vi "Send Libraries.vi"(8 "error in (no error)":errorcluster, 11 "Kasli Wrapper 2.0 in":refnum<class "Kasli Wrapper 2.0.lvclass">=refnum) -> (0 "error out":errorcluster, 3 "Kasli Wrapper 2.0 out":refnum<class "Kasli Wrapper 2.0.lvclass">)   [LabVIEW 2020, in "CIRCUS_uServices.lvlib" / "Kasli Wrapper 2.0.lvlib" / "Kasli Wrapper 2.0.lvclass"]
uses:
  Kasli Wrapper 2.0.lvclass
  TALOS/TALOS_PPL.lvlibp/Father of all uServices/Father of all uServices/Father of all uServices.lvclass
  Kasli Wrapper 2.0.lvlib
  Kasli/Kasli.lvclass
  C:/Users/marco/Documents/GitHub_Lab/CIRCUS/TALOS/TALOS_PPL.lvlibp/Ancestor/Ancestor/Ancestor.lvclass
  C:/Users/marco/Documents/GitHub_Lab/CIRCUS/TALOS/Actor Framework.lvlibp/1abvi3w/vi.lib/ActorFramework/Actor/Actor.lvclass
  C:/Users/marco/Documents/GitHub_Lab/CIRCUS/TALOS/TALOS_PPL.lvlibp/Father of all uServices/Father of all uServices/Father of all uServices.lvclass
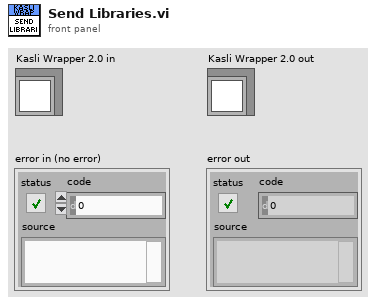
[diagram p1: front panel]
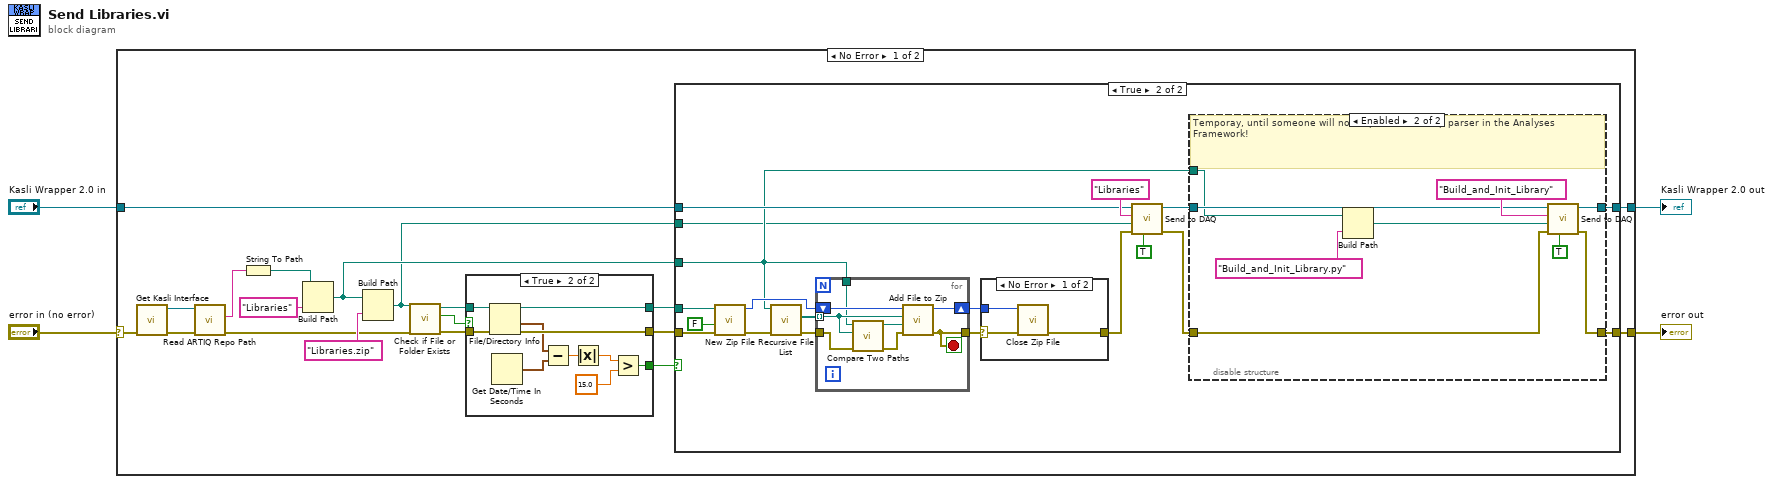
[diagram p0: block diagram]
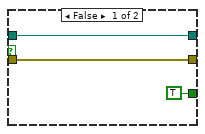
[diagram p2: hidden frame]
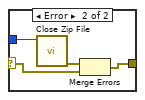
[diagram p5: hidden frame]
diagram:
  n1 = case shown="No Error" "error in (no error)" {
    selector: "error in (no error)" -> [w19 w84]
    tunnel: [w17 w84] -> w4
    tunnel: "Kasli Wrapper 2.0 in" -> [w18 w85]
    tunnel: [w16 w85] -> w1
    frame No Error {
      n2 = call "Get Kasli Interface.vi"("error in"=w19) -> ("error out"=w13:errorcluster, "Kasli Interface"=w14:refnum<class "Kasli.lvclass">)  [unwired: 9 in]
      n3 = call-dynamic "Read ARTIQ Repo Path.vi"("error in (no error)"=w13, "Kasli in"=w14) -> ("error out"=w11:errorcluster, "ARTIQ Repo Path"=w20:string)  [unwired: 7 in, 1 out]
      n4 = String To Path(string=w20) -> (path=w21:path)
      n5 = Build Path(base path=w21, name or relative path="Libraries" ("Parameter Name")) -> (appended path=w15:path)
      n6 = Build Path(base path=w15, name or relative path="Libraries.zip" ("Parameter Name")) -> (appended path=w12:path)
      n7 = call <vilib>:"Check if File or Folder Exists.vi"("error in (no error)"=w11, "path"=w12) -> ("error out"=w8:errorcluster, "file or folder exists?"=w10:bool, "dup path"=w9:path)  [unwired: 7 in]
      n8 = case shown="True" w10 {
        tunnel: w9 -> [w26 w35]
        tunnel: w8 -> [w25 w36]
        tunnel: [w26 w34] -> w7
        tunnel: [w25 w33] -> w6
        tunnel: [TRUE w27] -> w5
        frame False {
        }
        frame True {
          n9 = File/Directory Info(path=w35, error in=w36) -> (path out=w34:path, last mod=w32:timestamp, error out=w33:errorcluster)  [unwired: 4 out]
          n10 = Get Date/Time In Seconds() -> (seconds since 1Jan1904=w31:timestamp)
          n11 = Subtract(x=w32, y=w31) -> (x-y=w30:dbl)
          n12 = Absolute Value(x=w30) -> (abs(x)=w29:dbl)
          n13 = Greater?(x=w29, y=15.0) -> (0:w27:bool)
        }
      }
      n14 = case shown="True" w5 {
        tunnel: w18 -> [w38 w47]
        tunnel: [w37 w44] -> w17
        tunnel: [w38 w43] -> w16
        tunnel: w15 -> [_ w42]
        tunnel: w12 -> [_ w41]
        tunnel: w6 -> [w37 w40]
        tunnel: w7 -> [_ w39]
        frame False {
        }
        frame True {
          n15 = call <vilib>:"New Zip File.vi"("error in (no error)"=w40, "confirm overwrite? (F)"=FALSE, "target"=w39) -> ("error out"=w53:errorcluster, "zip file out"=w54:i64)  [unwired: 2 in, 1 out]
          n16 = call <vilib>:"Recursive File List.vi"("error in (no error)"=w53, "Folder Path"=w42) -> ("error out"=w55:errorcluster, "All Files in Dir"=w56:path[])  [unwired: 5 in, 3 out]
          n17 = for {
            tunnel: w55 -> [w60]
            tunnel: w56 -> [w59] mode=indexing
            tunnel: [w63] -> w51
            shift-right: [w64] -> w57
            shift-left: w54 -> [w65]
            tunnel: w42 -> [w58]
            stop <- w63 stop-if-true
            n18 = call <vilib>:"Compare Two Paths.vi"("error in (no error)"=w60, "Path 2"=w59, "Path 1"=w58) -> ("error out"=w61:errorcluster, "Relative Path from 1 to 2"=w62:path)  [unwired: 5 in, 2 out]
            n19 = call <vilib>:"Add File to Zip.vi"("error in (no error)"=w61, "destination path in zip"=w62, "source file path"=w59, "zip file in"=w65) -> ("error out"=w63:errorcluster, "zip file out"=w64:i64)  [unwired: 6 in]
          }
          n20 = case shown="No Error" w51 {
            selector: w51 -> [w78 w83]
            tunnel: w57 -> [w79 w80]
            tunnel: [w77 w81] -> w48
            frame No Error {
              n21 = call <vilib>:"Close Zip File.vi"("error in (no error)"=w78, "zip file in"=w79) -> ("error out"=w77:errorcluster)  [unwired: 5 in]
            }
            frame Error {
              n22 = call <vilib>:"Close Zip File.vi"("zip file in"=w80) -> ("error out"=w82:errorcluster)  [unwired: 6 in]
              n23 = Merge Errors(w82, w83) -> (w81:errorcluster)
            }
          }
          n24 = call "Send to DAQ.vi"("File?"=TRUE, "error in (no error)"=w48, "Data"=w41, "Data Name"="Libraries", "Father of all uServices in"=w47) -> ("error out"=w45:errorcluster, "Father of all uServices out"=w46:refnum<class "Father of all uServices.lvclass">)  [unwired: 5 in]
          n25 = disable-structure shown="Enabled" {
            disable-tunnel: w46 -> [w66 w73]
            disable-tunnel: w45 -> [w67 w69]
            disable-tunnel: [w67 w68] -> w44
            disable-tunnel: [w66 w74] -> w43
            disable-tunnel: w42 -> [_ w71]
            frame Disabled {
              # "The fiucha!"
            }
            frame Enabled {
              # "Temporay, until someone will not implement the zip parser in the Analyses Framework!"
              n26 = Build Path(base path=w71, name or relative path="Build_and_Init_Library.py" ("Parameter Name")) -> (appended path=w70:path)
              n27 = call "Send to DAQ.vi"("File?"=TRUE, "error in (no error)"=w69, "Data"=w70, "Data Name"="Build_and_Init_Library", "Father of all uServices in"=w73) -> ("error out"=w68:errorcluster, "Father of all uServices out"=w74:refnum<class "Father of all uServices.lvclass">)  [unwired: 5 in]
            }
          }
        }
      }
    }
    frame Error {
    }
  }
  "error out" <- w4
  "Kasli Wrapper 2.0 out" <- w1
